vi "libdaq_device_rename_byname.vi"(0 "error in (no error)":errorcluster, 3 "device_name":string, 5 "newname":string) -> (14 "error out":errorcluster)   [LabVIEW 2010, in "libdaqVI.lvlib"]
doc: "通过设备名称对设备进行重命名操作"
uses:
  libdaqVI.lvlib
  dll/daqlib.dll
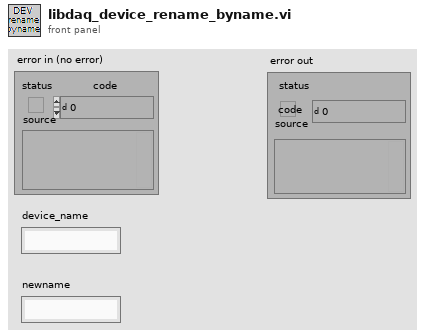
[diagram p1: front panel]
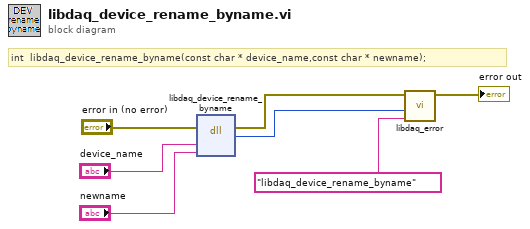
[diagram p0: block diagram]
diagram:
  # "int  libdaq_device_rename_byname(const char * device_name,const char * newname);"
  n1 = dll-call lib="E:/Product/Example/DAQ-USB3212/Labview/labview_2010/libdaqVI/dll/daqlib.dll" fn="libdaq_device_rename_byname"(error in="error in (no error)", "device_name"="device_name", "newname"="newname") -> (error out=w4:errorcluster, "return type"=w2:i32)  [unwired: 4 in, 1 out]
  n2 = call "libdaq_error.vi"("error source"="libdaq_device_rename_byname", "error code"=w2, "错误输入（无错误）"=w4) -> ("错误输出"=→"error out":errorcluster)  [unwired: 8 in]
